vi "iWorx - Periodic Motion Lab.vi"() -> ()   [LabVIEW 2012]
doc: "This VI is designed to work with myDAQ and the iWorx Light Sensor & Laser to measure periodic tasks."
uses:
  <vilib>/DAQmx/read.llb/DAQmx Read (Analog 1D Wfm NChan NSamp).vi
  <vilib>/DAQmx/create/channels.llb/DAQmx Create Channel (AI-Voltage-Basic).vi
  <vilib>/DAQmx/configure/timing.llb/DAQmx Timing (Sample Clock).vi
  <vilib>/DAQmx/miscellaneous.llb/DAQmx Fill In Error Info.vi
panel:
  in  "Number of Edges to store":u8=10 min=2
  in  "Channel":u16(ring) items=["Channel 1", "Channel 2"]
  out "Rising Edge Delta t":dbl[](array[numeric]) format="%.3fs"
  out "Beam Break Time":dbl[](array[numeric]) format="%.3fs"
  in  "Threshold":dbl format="%.2f V"
  out "Raw Signal":dbl(knob) scale=-5.0..5.0
  in  "Set Up":bool
  in  "Pause Button":bool
  in  "Snapshot":bool
  in  "stop":bool
  out "Waveform Chart":waveform(dbl)(graph)
  in  "Clear Chart":bool
  in  "Open Log":bool
  # "Periodic Motion Lab"
  # "Sensor Input"
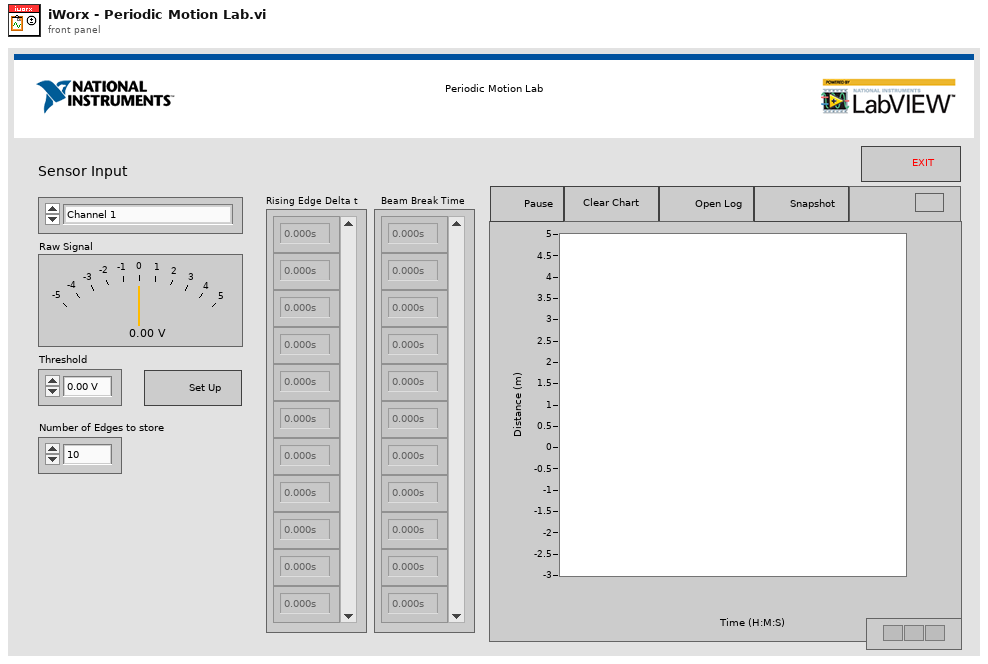
[diagram p1: front panel]
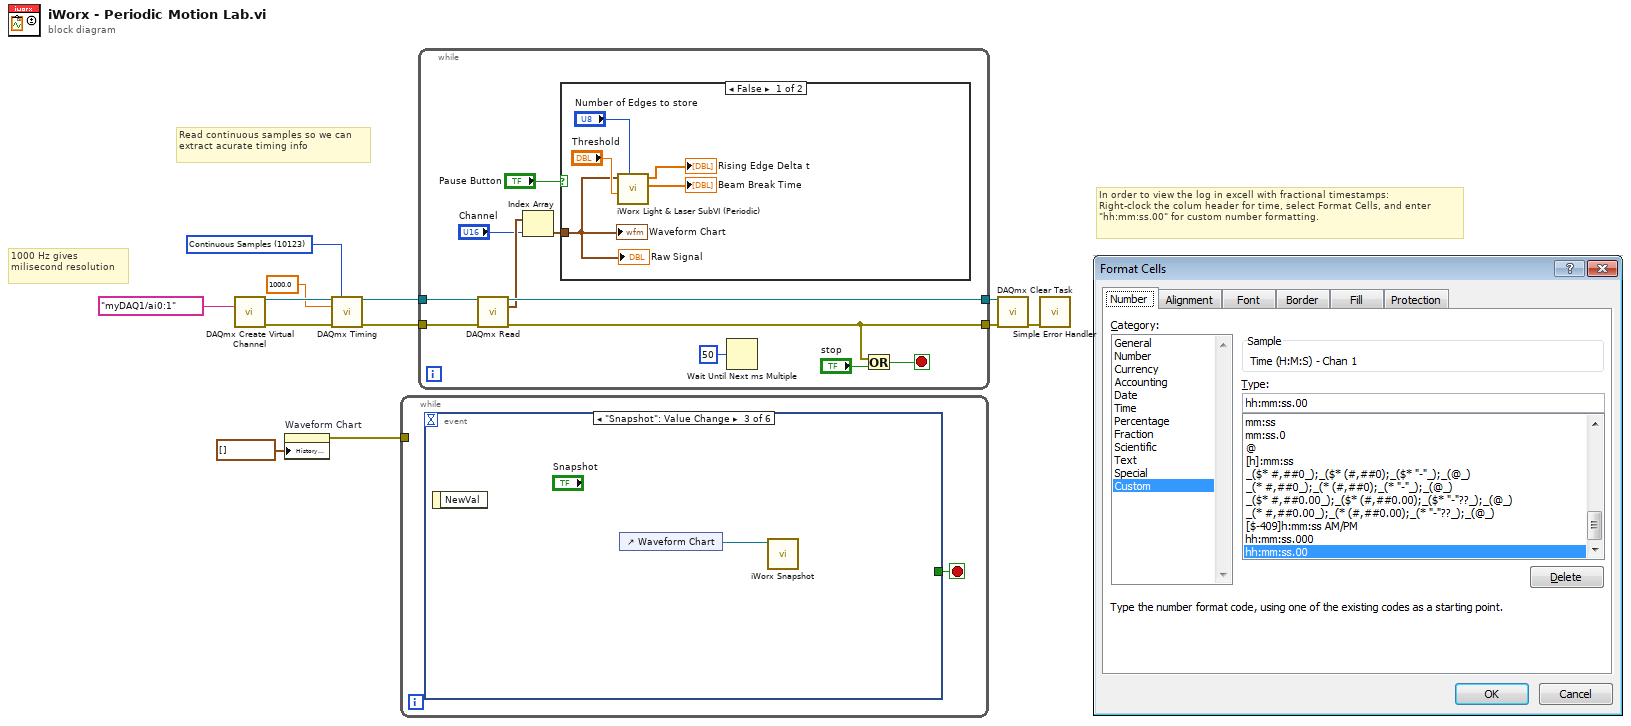
[diagram p0: block diagram]
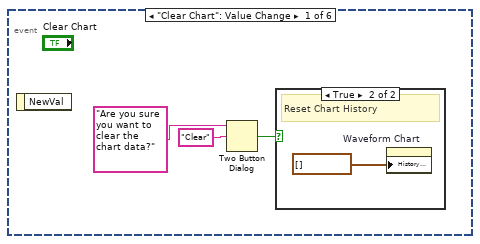
[diagram p2: hidden frame]
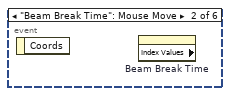
[diagram p4: hidden frame]
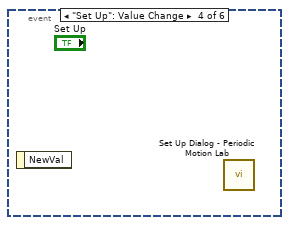
[diagram p5: hidden frame]
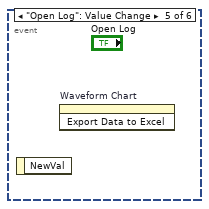
[diagram p6: hidden frame]
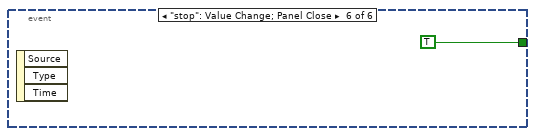
[diagram p7: hidden frame]
diagram:
  w2 = 10123 items=["Finite Samples"=10178, "Continuous Samples"=10123, "Hardware Timed Single Point"=12522] ("sample mode")
  # "1000 Hz gives milisecond resolution"
  # "Read continuous samples so we can extract acurate timing info"
  # "In order to view the log in excell with fractional timestamps: \nRight-clock the colum header for time, select Format Cells, and enter \"hh:mm:ss.00\" for custom number formatting."
  n1 = call-poly <vilib>:"DAQmx Create Virtual Channel.vi"("physical channels"=tag "myDAQ1/ai0:1") -> ("task out"=w7:refnum<k21>, "error out"=w4:errorcluster)  [unwired: 13 in]
  n2 = property on="Waveform Chart" class="WFChart (strict)"("History Data"=waveform(dbl)[] []) -> (error out=w9:errorcluster)  [unwired: 2 in, 1 out]
  n3 = call-poly <vilib>:"DAQmx Timing.vi"("task/channels in"=w7, "sample mode"=w2, "rate"=1000.0, "error in"=w4) -> ("task out"=w6:refnum<k21>, "error out"=w5:errorcluster)  [unwired: 10 in]
  n4 = while {
    tunnel: w9 -> [_]
    stop <- w13 stop-if-true
    n5 = event shown="[2] \"Snapshot\": Value Change" {
      selector: _ -> [_ _ _ _ _ _]
      dyn-events: _ -> [_ _ _ _ _ _]
      timeout: _ -> [_ _ _ _ _ _]
      tunnel: [_ _ _ _ _ TRUE] -> w13
      event "Clear Chart": Value Change {
        n6 = event-data() -> ()  [unwired: 1 in, 1 out]
        n7 = Two Button Dialog(message="Are you sure you want to clear the chart data?", 2:"Clear" ("T button name (\"OK\")")) -> (T button?=w15:bool)  [unwired: 1 in]
        n8 = case shown="True" w15 {
          frame False {
            # "Dialog canceled"
          }
          frame True {
            # "Reset Chart History"
            n9 = property on="Waveform Chart" class="WFChart (strict)"("History Data"=waveform(dbl)[] []) -> ()  [unwired: 2 in, 2 out]
          }
        }
      }
      event "Beam Break Time": Mouse Move {
        n10 = event-data() -> ()  [unwired: 1 in, 1 out]
        n11 = property on="Beam Break Time" class="Arr (strict)" props=["Index Values"]() -> ()  [unwired: 2 in, 3 out]
      }
      event "Snapshot": Value Change {
        n12 = event-data() -> ()  [unwired: 1 in, 1 out]
        n13 = control-ref of="Waveform Chart"() -> (w18:refnum<vi>)
        n14 = call "iWorx Snapshot.vi"("WaveformChart in"=w18) -> ()  [unwired: 10 in, 1 out]
      }
      event "Set Up": Value Change {
        n15 = event-data() -> ()  [unwired: 1 in, 1 out]
        n16 = call "Set Up Dialog - Periodic Motion Lab.vi"() -> ()  [unwired: 12 in]
      }
      event "Open Log": Value Change {
        n17 = event-data() -> ()  [unwired: 1 in, 1 out]
        n18 = invoke on="Waveform Chart" class="WFChart (strict)" method="Export Data to Excel"() -> ()  [unwired: 3 in, 3 out]
      }
      event "stop": Value Change; Panel Close {
        n19 = event-data() -> ()  [unwired: 1 in, 3 out]
      }
    }
  }
  n20 = while {
    tunnel: w6 -> [w29]
    tunnel: [w24] -> w12
    tunnel: w5 -> [w28]
    tunnel: [w26] -> w11
    stop <- w27 stop-if-true
    n21 = call-poly <vilib>:"DAQmx Read.vi"("task/channels in"=w29, "error in"=w28) -> ("task out"=w24:refnum<k21>, "data"=w22:waveform(dbl)[], "error out"=w26:errorcluster)  [unwired: 11 in]
    n22 = Index Array(array=w22, index="Channel") -> (element=w21:waveform(dbl))
    n23 = case shown="False" "Pause Button" {
      tunnel: w21 -> [w34 _]
      frame False {
        n24 = call "iWorx Light & Laser SubVI (Periodic).vi"("# of Timestamps to store (10)"="Number of Edges to store", "Threshold"="Threshold", "Waveform"=w34) -> ("Beam Break Durration (s)"=→"Beam Break Time":dbl[], "Rising Edge Delta t (s)"=→"Rising Edge Delta t":dbl[])  [unwired: 5 in, 2 out]
        "Waveform Chart" <- w34
        "Raw Signal" <- w34
      }
      frame True {
      }
    }
    n25 = Wait Until Next ms Multiple(millisecond multiple=u32 50) -> ()  [unwired: 1 out]
    n26 = Or(x=w26, y="stop") -> (x .or. y?=w27:bool)
  }
  n27 = call <vilib>:"DAQmx Clear Task.vi"("task in"=w12, "error in"=w11) -> ("error out"=w8:errorcluster)  [unwired: 13 in]
  n28 = call <vilib>:"Simple Error Handler.vi"("error in (no error)"=w8) -> ()  [unwired: 4 in, 5 out]
